vi "AutoModeDynamics.vi"(8 "Timer Limit":u32, 9 "SelectFLaser":bool=TRUE, 10 "Stripe Limit":u32, 11 "Laser Readings":T1) -> (0 "Rip Cord Out?":bool, 1 "Timer Expired?":bool, 2 "Stripe Limit Exceeded?":bool, 3 "Brake Condition Reached?":bool, 4 "Timer Value(s)":u32, 6 "Stripe Count":u32)   [LabVIEW 2017]
uses:
  Type Defs/allLaserReadings.ctl
  Type Defs/laserReading.ctl
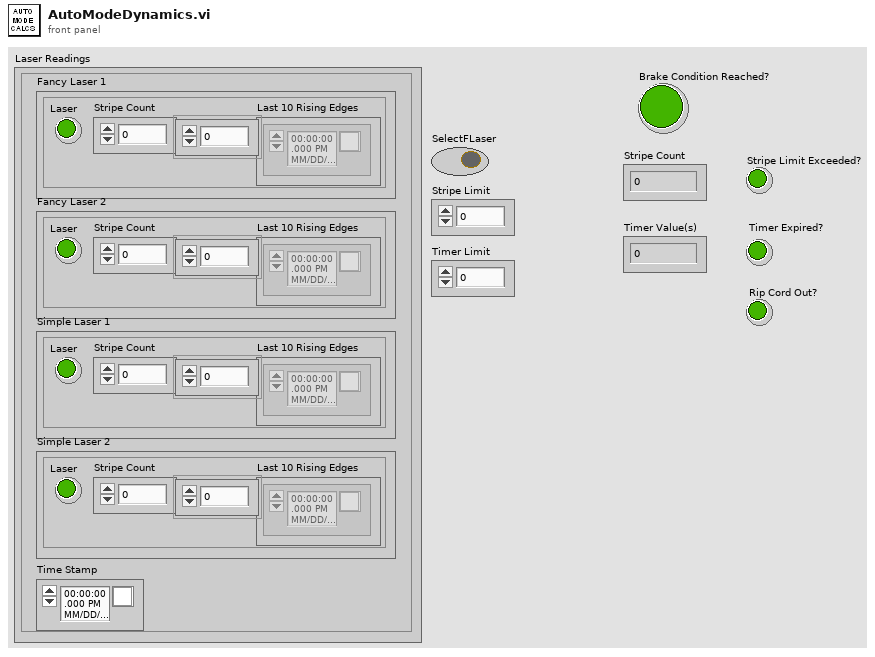
[diagram p1: front panel]
types:
  T1 = typedef "allLaserReadings.ctl" = cluster{"Fancy Laser 1":T2, "Fancy Laser 2":T2, "Simple Laser 1":T2, "Simple Laser 2":T2, "Time Stamp":timestamp}
  T2 = typedef "laserReading.ctl" = cluster{"Laser":bool, "Stripe Count":u32, "Last 10 Rising Edges":timestamp[]}
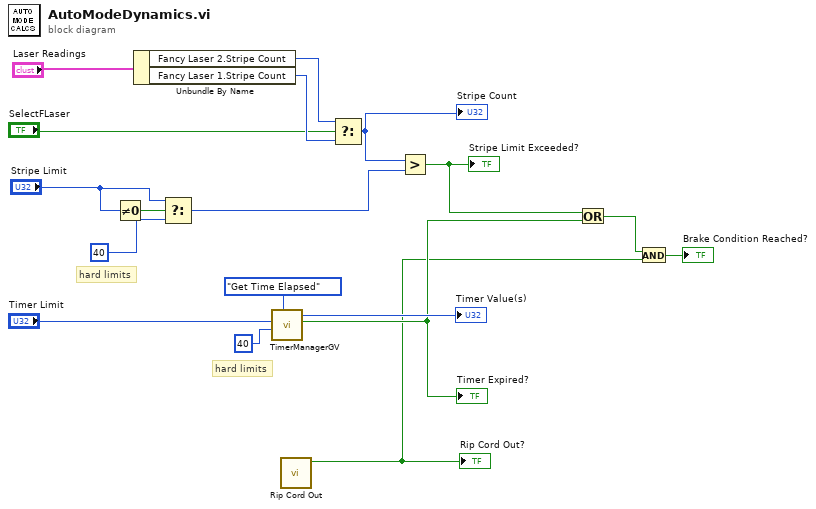
[diagram p0: block diagram]
diagram:
  # "hard limits"
  # "hard limits"
  n1 = Not Equal To 0?(x="Stripe Limit") -> (x != 0?=w4:bool)
  n2 = Unbundle By Name("Laser Readings") -> ("Fancy Laser 2.Stripe Count"=w13:u32, "Fancy Laser 1.Stripe Count"=w12:u32)
  n3 = Select(t="Stripe Limit", s=w4, f=u32 40) -> (s? t:f=w2:u32)
  n4 = call "TimerManagerGV.vi"("Command"=enum16{"Get Time Elapsed", "Start Timer"}."Get Time Elapsed", "Hard Limit (s)"=u32 40, "Time to Wait (s)"="Timer Limit") -> ("Timer Expired?"=w8:bool, "Timer Value(s)"=→"Timer Value(s)":u32)  [unwired: 7 in]
  "Timer Expired?" <- w8
  n5 = call "Rip Cord Out"() -> ("Rip Cord Out?"=w6:bool)  [unwired: 11 in]
  "Rip Cord Out?" <- w6
  n6 = Select(t=w13, s="SelectFLaser", f=w12) -> (s? t:f=w10:u32)
  "Stripe Count" <- w10
  n7 = Greater?(x=w10, y=w2) -> (0:w9:bool)
  "Stripe Limit Exceeded?" <- w9
  n8 = Or(x=w9, y=w8) -> (x .or. y?=w7:bool)
  n9 = And(x=w7, y=w6) -> (x .and. y?=→"Brake Condition Reached?":bool)
